vi "Enter Program Mode.vi"(4 "error in (no error)":errorcluster, 6 "Program Number (1)":i32=1 min=1 max=100, 7 "VISA resource name":refnum<visa-resource-name>) -> (0 "error out":errorcluster, 3 "VISA resource name out":refnum<visa-resource-name>)   [LabVIEW 2020, in "Newport ESP301.lvlib"]
doc: "This command sets the controller in programming mode. All the commands following this one will not be executed immediately but stored in memory as part of program number xx. To exit program entry mode and return to immediate mode, use QP command.\nPrograms can be entered in any order. If a program already exists then it must be first deleted using XX command.\nNote:\nPrograms are automatically stored into non-volatile memory when created."
uses:
  Newport ESP301.lvlib
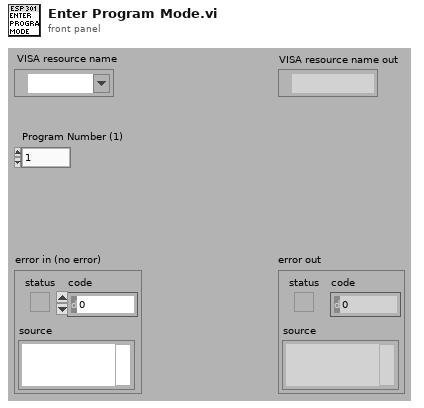
[diagram p1: front panel]
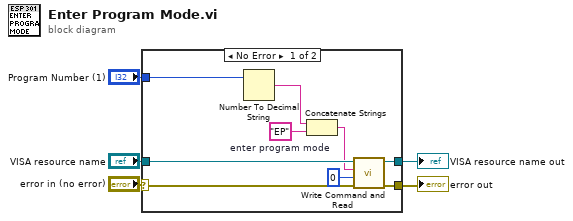
[diagram p0: block diagram]
diagram:
  n1 = case shown="No Error" "error in (no error)" {
    selector: "error in (no error)" -> [w11 w16]
    tunnel: [w13 w16] -> w5
    tunnel: "VISA resource name" -> [w14 w15]
    tunnel: [w12 w15] -> w4
    tunnel: "Program Number (1)" -> [w7 _]
    frame No Error {
      w10 = "EP"  # enter program mode
      n2 = Number To Decimal String(number=w7) -> (decimal integer string=w9:string)  [unwired: 1 in]
      n3 = Concatenate Strings(w9, w10) -> (w8:string)
      n4 = call "Write Command and Read.vi"("error in (no error)"=w11, "Bytes to read (100)"=u32 0, "Command"=w8, "VISA resource name"=w14) -> ("error out"=w13:errorcluster, "VISA resource name out"=w12:refnum<visa-resource-name>)  [unwired: 3 in, 1 out]
    }
    frame Error {
    }
  }
  "error out" <- w5
  "VISA resource name out" <- w4
